vi "Boolean.vi"() -> (0 "error out":errorcluster, 3 "Passed?":bool)   [LabVIEW 2009]
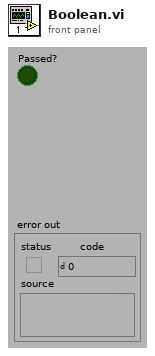
[diagram p1: front panel]
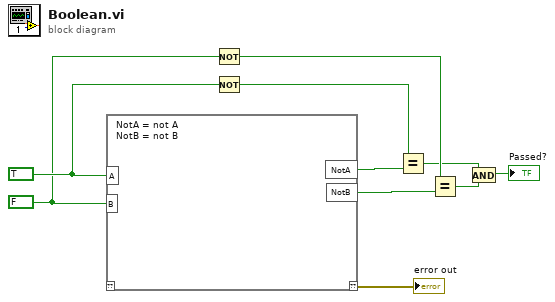
[diagram p0: block diagram]
diagram:
  w5 = FALSE ("Boolean")
  w8 = TRUE ("Boolean")
  n1 = script code="NotA = not A\nNotB = not B"("A"=w8, "B"=w5) -> ("??"=→"error out":errorcluster, "NotA"=w9:bool, "NotB"=w6:bool)  [unwired: 1 in]
  n2 = Not(x=w5) -> (.not. x?=w4:bool)
  n3 = Not(x=w8) -> (.not. x?=w7:bool)
  n4 = Equal?(x=w7, y=w9) -> (x = y?=w3:bool)
  n5 = Equal?(x=w4, y=w6) -> (x = y?=w2:bool)
  n6 = And(x=w3, y=w2) -> (x .and. y?=→"Passed?":bool)
